vi "Average_Column_Values.vi"(1 "Present Values":string[][](array[string]), 2 "Present Channels":string[](array[string]), 3 "Channel operations":string[](array[string]), 4 "Channel names for operations":string[](array[string])) -> (0 "Desired Row values":string[](array[string]))   [LabVIEW 2010]
uses:
  <vilib>/Analysis/NI_AALBase.lvlib
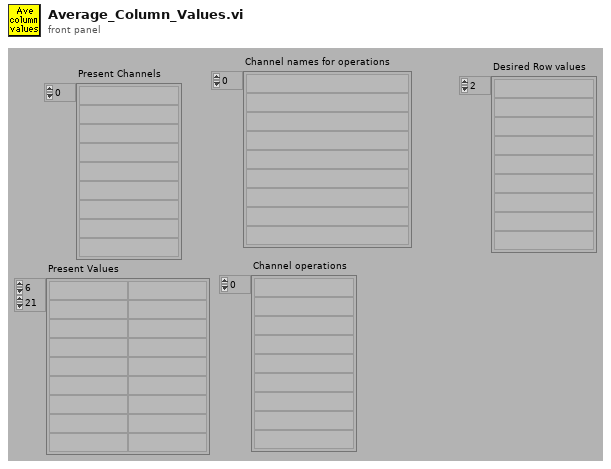
[diagram p1: front panel]
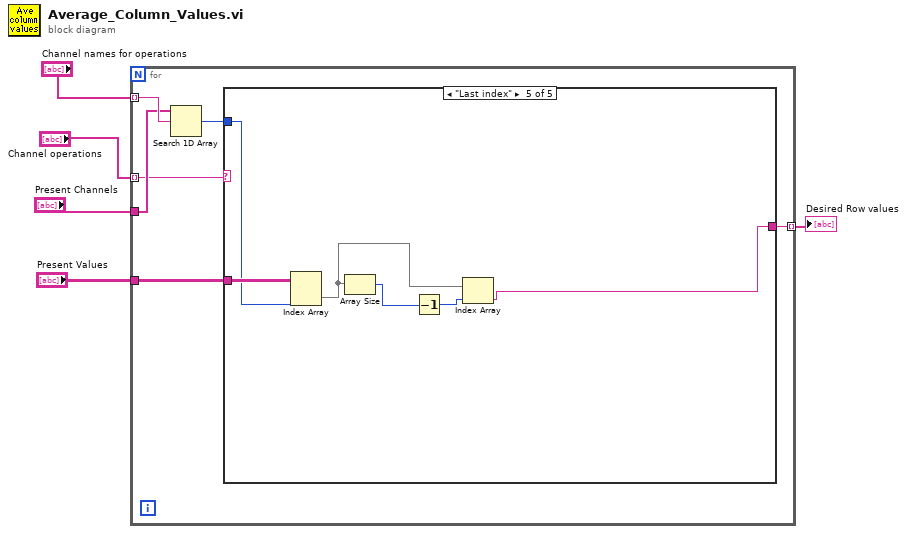
[diagram p0: block diagram]
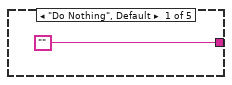
[diagram p2: hidden frame]
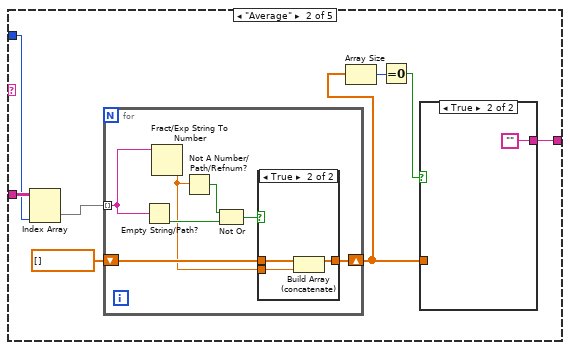
[diagram p3: hidden frame]
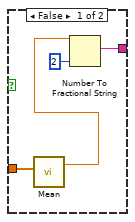
[diagram p4: hidden frame]
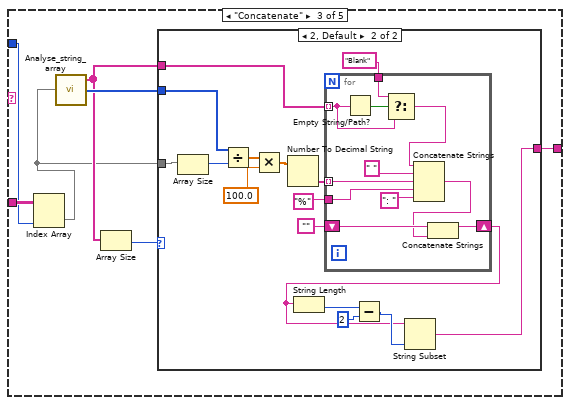
[diagram p6: hidden frame]
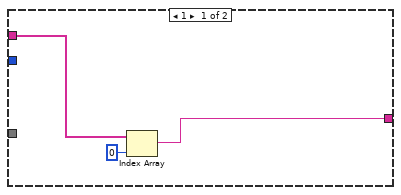
[diagram p7: hidden frame]
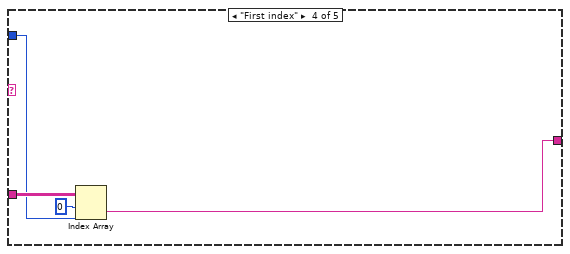
[diagram p8: hidden frame]
diagram:
  n1 = for {
    tunnel: "Channel names for operations" -> [w11] mode=indexing
    tunnel: "Present Channels" -> [w10]
    tunnel: "Channel operations" -> [w9] mode=indexing
    tunnel: "Present Values" -> [w8]
    tunnel: [w6] -> w3 mode=indexing
    n2 = Search 1D Array(1D array=w10, element=w11) -> (index of element=w7:i32)  [unwired: 1 out]
    n3 = case shown="\"Last index\"" w9 {
      tunnel: w8 -> [_ w20 w43 w77 w83]
      tunnel: w7 -> [_ w19 w42 w76 w82]
      tunnel: ["" w17 w41 w74 w78] -> w6
      frame "Do Nothing", Default {
      }
      frame "Average" {
        n4 = Index Array(array=w20, index (col)=w19) -> (element=w18:string[])  [unwired: 1 in]
        n5 = for {
          tunnel: w18 -> [w32] mode=indexing
          shift-right: [w28] -> w15
          shift-left: dbl[] [] -> [w27]
          n6 = Empty String/Path?(string/path=w32) -> (empty?=w30:bool)
          n7 = Fract/Exp String To Number(string=w32) -> (number=w26:dbl)  [unwired: 4 out]
          n8 = Not A Number/Path/Refnum?(number/path/refnum=w26) -> (NaN/Path/Refnum?=w31:bool)
          n9 = Not Or(1:w30, 2:w31) -> (0:w29:bool)
          n10 = case shown="True" w29 {
            tunnel: [w33 w34] -> w28
            tunnel: w27 -> [w33 w36]
            tunnel: w26 -> [_ w35]
            frame False {
            }
            frame True {
              n11 = Build Array (concatenate)(w36, w35) -> (w34:dbl[])
            }
          }
        }
        n12 = Array Size(array=w15) -> (size(s)=w14:i32)
        n13 = Equal To 0?(x=w14) -> (x = 0?=w13:bool)
        n14 = case shown="True" w13 {
          tunnel: [w23 ""] -> w17
          tunnel: w15 -> [w22 _]
          frame False {
            n15 = call <vilib>:"Mean.vi"("X"=w22) -> ("mean"=w21:dbl)  [unwired: 1 out]
            n16 = Number To Fractional String(number=w21, precision (6)=i16 2) -> (F-format string=w23:string)  [unwired: 2 out]
          }
          frame True {
          }
        }
      }
      frame "Concatenate" {
        n17 = Index Array(array=w43, index (col)=w42) -> (element=w37:string[])  [unwired: 1 in]
        n18 = call "Analyse_string_array.vi"("String array"=w37) -> ("Unique strings"=w39:string[], "Frequency"=w40:i32[])  [unwired: 1 out]
        n19 = Array Size(array=w39) -> (size(s)=w38:i32)
        n20 = case shown="2, Default" w38 {
          tunnel: [w45 w47] -> w41
          tunnel: w40 -> [_ w56]
          tunnel: w39 -> [w44 w55]
          tunnel: w37 -> [_ w52]
          frame 1 {
            n21 = Index Array(array=w44, index=0) -> (element=w45:string)
          }
          frame 2, Default {
            n22 = Array Size(array=w52) -> (size(s)=w53:i32)
            n23 = Divide(x=w56, y=w53) -> (x/y=w61:dbl[])
            n24 = Multiply(x=w61, y=100.0) -> (x*y=w58:dbl[])
            n25 = Number To Decimal String(number=w58) -> (decimal integer string=w57:string[])  [unwired: 1 out]
            n26 = for {
              tunnel: w57 -> [w73] mode=indexing
              tunnel: "%" -> [w72]
              shift-right: [w70] -> w48
              shift-left: "" -> [w69]
              tunnel: w55 -> [w65] mode=indexing
              tunnel: "Blank" -> [w67]
              n27 = Empty String/Path?(string/path=w65) -> (empty?=w66:bool)
              n28 = Select(t=w67, s=w66, f=w65) -> (s? t:f=w64:string)
              n29 = Concatenate Strings(w64, " ", w73, w72, ": ") -> (w63:string)
              n30 = Concatenate Strings(w69, w63) -> (w70:string)
            }
            n31 = String Length(string=w48) -> (length=w51:i32)
            n32 = Subtract(x=w51, y=2) -> (x-y=w49:i32)
            n33 = String Subset(string=w48, length (rest)=w49) -> (substring=w47:string)  [unwired: 1 out]
          }
        }
      }
      frame "First index" {
        n34 = Index Array(array=w77, index (row)=0, index (col)=w76) -> (element=w74:string)
      }
      frame "Last index" {
        n35 = Index Array(array=w83, index (col)=w82) -> (element=w81:string[])  [unwired: 1 in]
        n36 = Array Size(array=w81) -> (size(s)=w80:i32)
        n37 = Decrement(x=w80) -> (x-1=w79:i32)
        n38 = Index Array(array=w81, index=w79) -> (element=w78:string)
      }
    }
  }
  "Desired Row values" <- w3
